vi "Day6.vi"(11 "Input":string="47|53\n97|13\n97|61\n97|47\n75|29\n61|13\n75|53\n29|13\n97|29\n53|29\n61|53\n97|53\n61|29\n47|13\n75|47\n97|75\n47|61\n75|61\n47|29\n75|13\n53|13") -> (3 "Result":i64)   [LabVIEW 2024]
uses:
  <userlib>/_OpenG.lib/string/string.llb/openg_string.lvlib
panel:
  out "Array":i64[][](array[numeric])
  out "element":string
  out "X":i32
  out "Y":i32
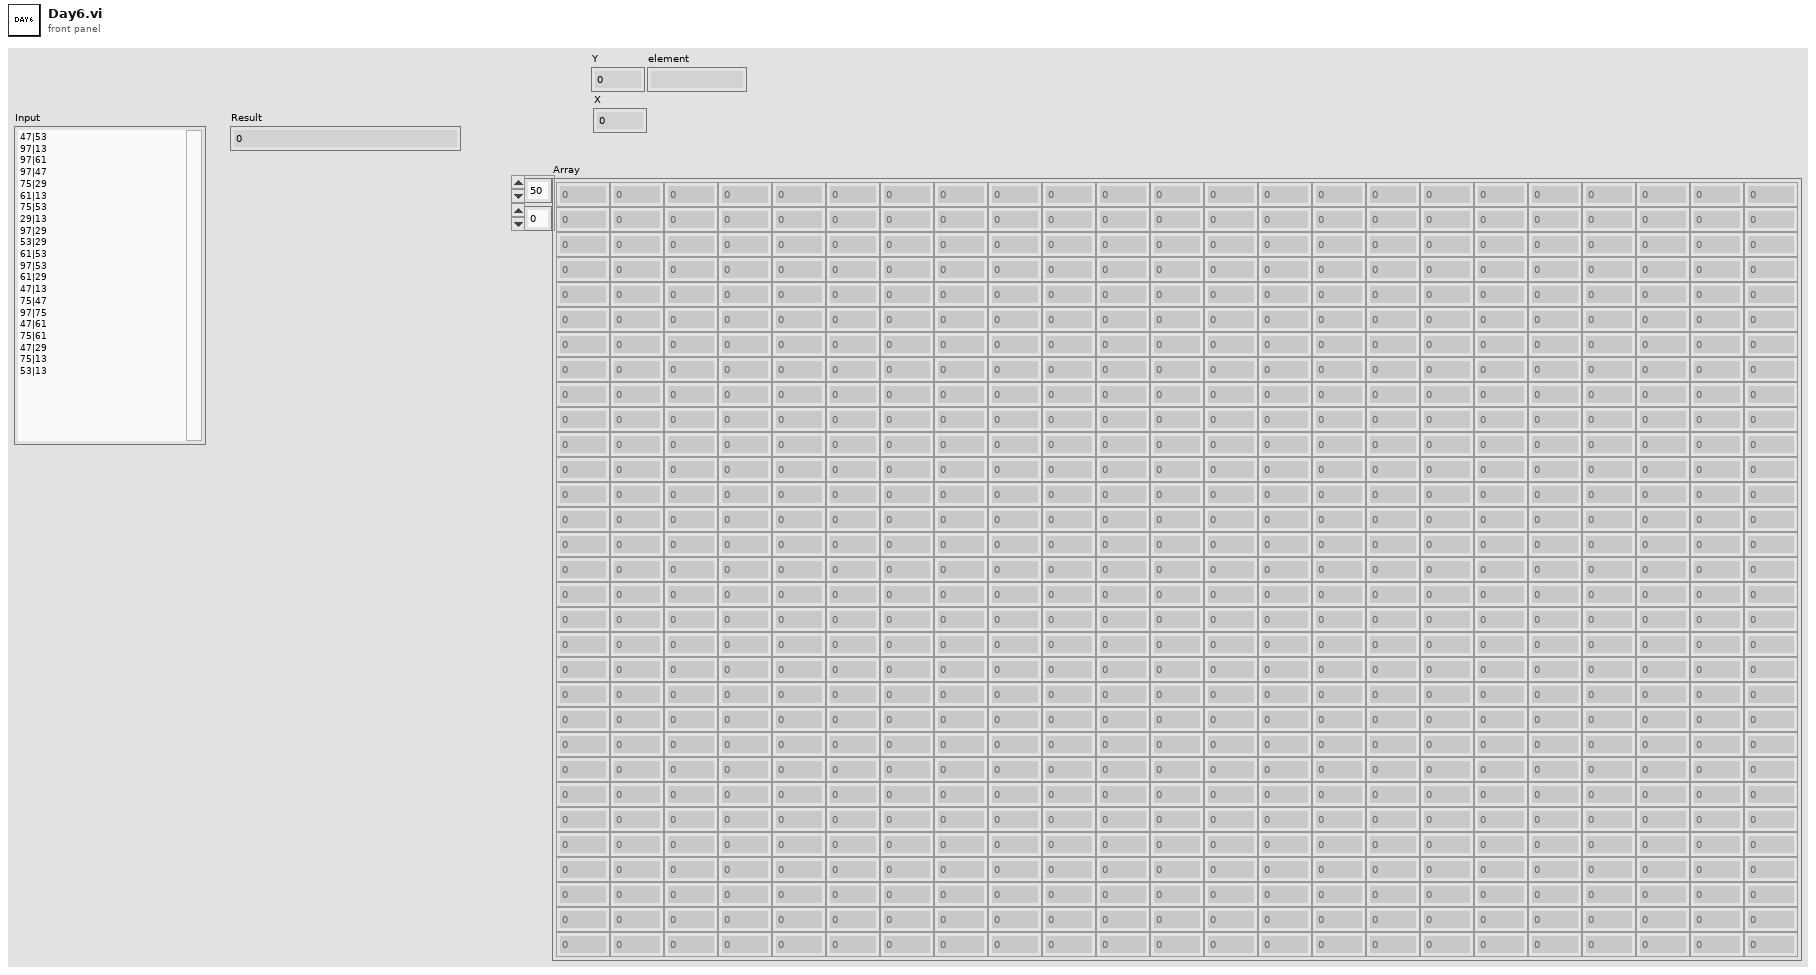
[diagram p1: front panel]
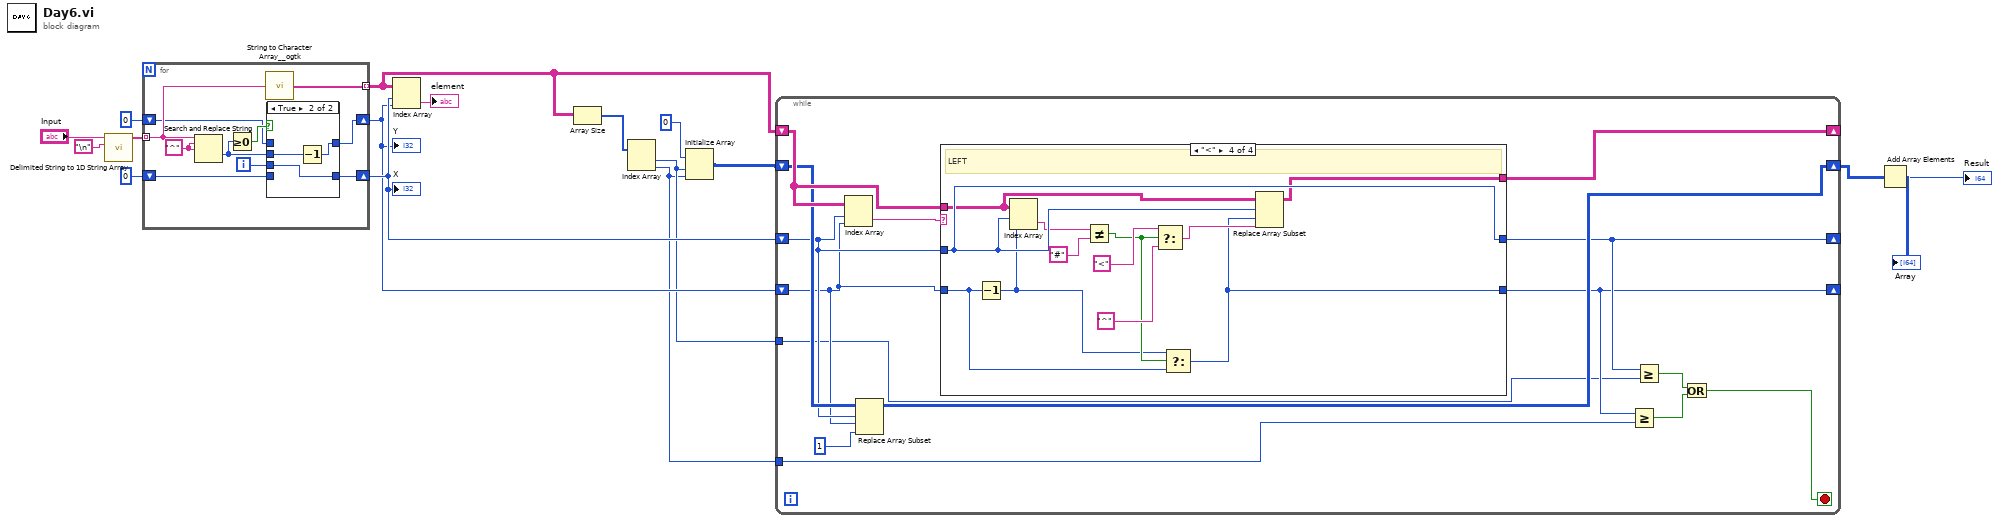
[diagram p0: block diagram]
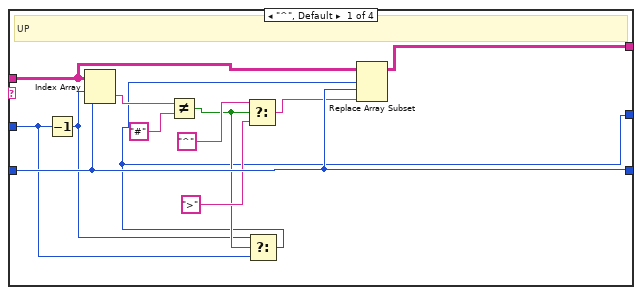
[diagram p2: hidden frame]
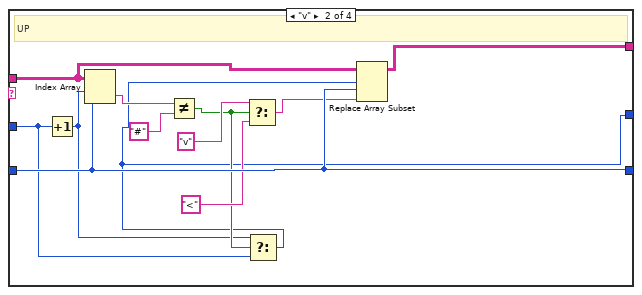
[diagram p3: hidden frame]
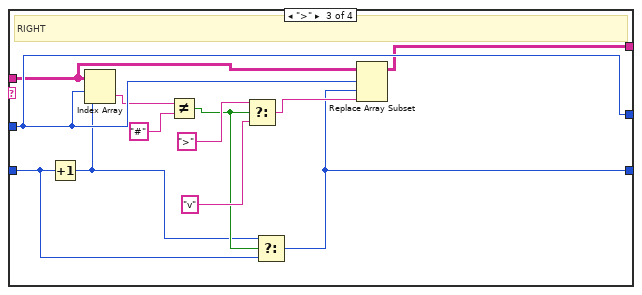
[diagram p4: hidden frame]
diagram:
  n1 = call <vilib>:"Delimited String to 1D String Array.vi"("delimiter"="\n", "delimited string"="Input") -> ("string array"=w14:string[])  [unwired: 9 in]
  n2 = for {
    tunnel: w14 -> [w25] mode=indexing
    tunnel: [w26] -> w10 mode=indexing
    shift-right: [w20] -> w4
    shift-left: 0 -> [w19]
    shift-right: [w18] -> w3
    shift-left: 0 ("offset past replacement") -> [w17]
    i -> [w21]
    w24 = "^" ("search string")
    n3 = Search and Replace String(input string=w25, search string=w24, replace string=w24) -> (offset past replacement=w22:i32)  [unwired: 5 in, 3 out]
    n4 = Greater Or Equal To 0?(x=w22) -> (x >= 0?=w23:bool)
    n5 = call <userlib>:"String to Character Array__ogtk.vi"("Input String"=w25) -> ("Character Array"=w26:string[])
    n6 = case shown="True" w23 {
      tunnel: w22 -> [_ w30]
      tunnel: w21 -> [_ w31]
      tunnel: [w28 w31] -> w20
      tunnel: w19 -> [w28 _]
      tunnel: [w27 w29] -> w18
      tunnel: w17 -> [w27 _]
      frame False {
      }
      frame True {
        n7 = Decrement(x=w30) -> (x-1=w29:i32)
      }
    }
  }
  "Y" <- w3
  "X" <- w4
  n8 = Index Array(array=w10, index (row)=w4, index (col)=w3) -> (element=→"element":string)
  n9 = Array Size(array=w10) -> (size(s)=w9:i32[])
  n10 = Index Array(array=w9) -> (element #1=w2:i32, element #2=w1:i32)  [unwired: 2 in]
  n11 = Initialize Array(i64 0, w2, w1) -> (w7:i64[][])
  n12 = while {
    shift-right: [w39] -> w6
    shift-left: w7 -> [w43]
    shift-right: [w35] -> _
    shift-left: w4 -> [w42]
    shift-right: [w34] -> _
    shift-left: w3 -> [w41]
    shift-right: [w44] -> _
    shift-left: w10 -> [w45]
    tunnel: w2 -> [w33]
    tunnel: w1 -> [w32]
    stop <- w36 stop-if-true
    n13 = Index Array(array=w45, index (row)=w42, index (col)=w41) -> (element=w46:string)
    n14 = Replace Array Subset(array=w43, new element=i64 1, index (row)=w42, index (col)=w41) -> (w39:i64[][])
    n15 = case shown="\"<\"" w46 {
      tunnel: w42 -> [w49 w61 w82 w94]
      tunnel: [w47 w59 w82 w94] -> w35
      tunnel: w41 -> [w55 w67 w72 w84]
      tunnel: [w55 w67 w71 w83] -> w34
      tunnel: w45 -> [w56 w68 w79 w91]
      tunnel: [w51 w63 w75 w87] -> w44
      frame "^", Default {
        # "UP"
        n16 = Decrement(x=w49) -> (x-1=w48:i32)
        n17 = Index Array(array=w56, index (row)=w48, index (col)=w55) -> (element=w58:string)
        n18 = Not Equal?(x=w58, y="#") -> (x != y?=w50:bool)
        n19 = Select(t="^", s=w50, f=">") -> (s? t:f=w52:string)
        n20 = Select(t=w48, s=w50, f=w49) -> (s? t:f=w47:i32)
        n21 = Replace Array Subset(array=w56, new element=w52, index (row)=w47, index (col)=w55) -> (w51:string[][])
      }
      frame "v" {
        # "UP"
        n22 = Increment(x=w61) -> (x+1=w60:i32)
        n23 = Index Array(array=w68, index (row)=w60, index (col)=w67) -> (element=w70:string)
        n24 = Not Equal?(x=w70, y="#") -> (x != y?=w62:bool)
        n25 = Select(t="v", s=w62, f="<") -> (s? t:f=w64:string)
        n26 = Select(t=w60, s=w62, f=w61) -> (s? t:f=w59:i32)
        n27 = Replace Array Subset(array=w68, new element=w64, index (row)=w59, index (col)=w67) -> (w63:string[][])
      }
      frame ">" {
        # "RIGHT"
        n28 = Increment(x=w72) -> (x+1=w73:i32)
        n29 = Index Array(array=w79, index (row)=w82, index (col)=w73) -> (element=w81:string)
        n30 = Not Equal?(x=w81, y="#") -> (x != y?=w74:bool)
        n31 = Select(t=">", s=w74, f="v") -> (s? t:f=w76:string)
        n32 = Select(t=w73, s=w74, f=w72) -> (s? t:f=w71:i32)
        n33 = Replace Array Subset(array=w79, new element=w76, index (row)=w82, index (col)=w71) -> (w75:string[][])
      }
      frame "<" {
        # "LEFT"
        n34 = Decrement(x=w84) -> (x-1=w85:i32)
        n35 = Index Array(array=w91, index (row)=w94, index (col)=w85) -> (element=w93:string)
        n36 = Not Equal?(x=w93, y="#") -> (x != y?=w86:bool)
        n37 = Select(t="<", s=w86, f="^") -> (s? t:f=w88:string)
        n38 = Select(t=w85, s=w86, f=w84) -> (s? t:f=w83:i32)
        n39 = Replace Array Subset(array=w91, new element=w88, index (row)=w94, index (col)=w83) -> (w87:string[][])
      }
    }
    n40 = Greater Or Equal?(x=w34, y=w32) -> (x >= y?=w37:bool)
    n41 = Greater Or Equal?(x=w35, y=w33) -> (x >= y?=w38:bool)
    n42 = Or(x=w38, y=w37) -> (x .or. y?=w36:bool)
  }
  "Array" <- w6
  n43 = Add Array Elements(numeric array=w6) -> (sum=→"Result":i64)
